vi "Write to Lights.vi"   [LabVIEW 2015]
uses:
  Common Code/Shooter State.ctl
  <vilib>/Rock Robotics/WPI/DriverStation/WPI_DriverStationRobotMode2.ctl
  <vilib>/Rock Robotics/WPI/DriverStation/WPI_DriverStationAllianceInfo.ctl
  Common Code/Utilities/TimeManager.vi
  Common Code/Change Detect.vi
  Common Code/Change Detect Boolean.vi
  Robot Global Data.vi
types:
  T1 = typedef "WPI_DriverStationAllianceInfo.ctl" = enum16{"Red", "Blue", "Invalid"}
  T2 = typedef "Shooter State.ctl" = enum16{"Idle", "Settle Ball", "Warmup", "Shooter Ready", "Shoot"}
  T3 = typedef "WPI_DriverStationRobotMode2.ctl" = enum16{"Autonomous Disabled", "Autonomous Enabled", "Teleop Disabled", "Teleop Enabled", "Disconnected", "Finish", "Test Disabled", "Test Enabled", "Emergency Stopped"}
  T4 = typedef "Shooter State Cluster.ctl" = cluster{"State":T2, "Left RPM":dbl, "Right RPM":dbl, "Shooter Ready?":bool, "Ball Loaded?":bool, "Current Angle":dbl, "Angle Motor Output":dbl, "Trigger Output":dbl, "Angle Ready?":bool, "RPM Ready?":bool, "Vision Ready?":bool, "Ball Loaded?":bool, "Mode":T5, "Shot Type":T6, "Pot Height":dbl, "Current Tripped Forward?":bool, "Current Tripped Backward?":bool, "Right Servo":i32, "Left Servo":i32, "IR Override":bool, "Intake Danger?":bool, "Intake Angle Ready?":bool}
  T5 = typedef "Shoot Modes Enum.ctl" = enum16{"Manual", "Auto"}
  T6 = typedef "Shot Type.ctl" = enum16{"Batter Shot", "Corner Shot", "Cleat Shot", "Vision Shot", "Deep Middle Shot"}
  T7 = typedef "WPI_AOChannelDevRef.ctl" = cluster{"DevStatus":errorcluster, "AO Channel":T8}
  T8 = typedef "WPI_AnalogOutputChannel.ctl" = enum8{"AO MXP 0", "AO MXP 1", "Invalid"}
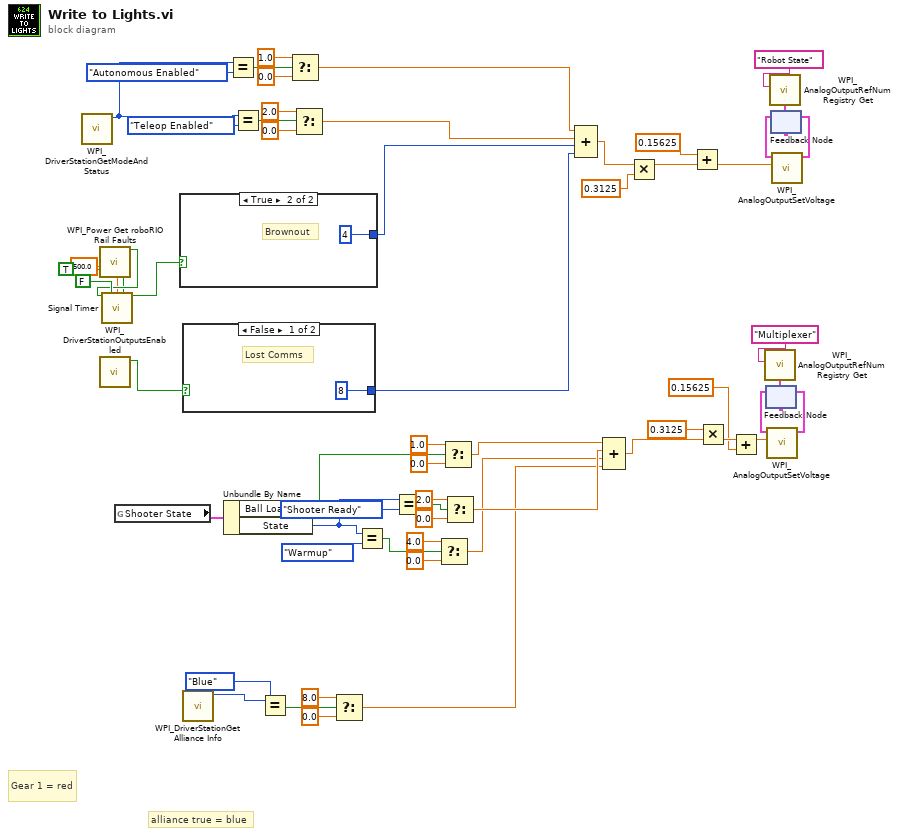
[diagram p0: block diagram]
diagram:
  # "alliance true = blue"
  # "Gear 1 = red"
  n1 = call <vilib>:"WPI_DriverStationGetModeAndStatus.vi"() -> ("Robot Mode"=w25:T3)  [unwired: 10 in, 1 out]
  n2 = call <vilib>:"WPI_Power Get roboRIO Rail Faults.vi"() -> ("Input Voltage Brown Out"=w50:bool)  [unwired: 10 in, 5 out]
  n3 = call <vilib>:"WPI_DriverStationOutputsEnabled.vi"() -> ("OutputsEnabled?"=w45:bool)  [unwired: 10 in, 1 out]
  n4 = call "Signal Timer.vi"("Input"=w50, "Edge"=FALSE, "Interval"=500.0, "Pull"=TRUE) -> ("Filtered Output"=w48:bool)  [unwired: 11 in]
  n5 = global read "Robot Global Data.vi" "Shooter State"() -> (w38:T4)
  n6 = case shown="True" w48 {
    tunnel: [_ 4] -> w44
    frame False {
    }
    frame True {
      # "Brownout"
    }
  }
  n7 = case shown="False" w45 {
    tunnel: [8 _] -> w43
    frame False {
      # "Lost Comms"
    }
    frame True {
    }
  }
  n8 = call <vilib>:"WPI_DriverStationGet Alliance Info.vi"() -> ("Alliance"=w7:T1)  [unwired: 10 in, 1 out]
  n9 = Unbundle By Name(w38) -> ("Ball Loaded?"=w35:bool, "State"=w36:T2)
  n10 = Equal?(x=w25, y=WPI_DriverStationRobotMode2."Autonomous Enabled") -> (x = y?=w23:bool)
  n11 = Equal?(x=w25, y=WPI_DriverStationRobotMode2."Teleop Enabled") -> (x = y?=w22:bool)
  n12 = Equal?(x=w7, y=WPI_DriverStationAllianceInfo."Blue") -> (x = y?=w5:bool)
  n13 = Select(t=1.0, s=w23, f=0.0) -> (s? t:f=w17:dbl)
  n14 = Select(t=2.0, s=w22, f=0.0) -> (s? t:f=w16:dbl)
  n15 = Select(t=8.0, s=w5, f=0.0) -> (s? t:f=w1:dbl)
  n16 = Equal?(x=w36, y=Shooter_State."Warmup") -> (x = y?=w29:bool)
  n17 = Equal?(x=w36, y=Shooter_State."Shooter Ready") -> (x = y?=w32:bool)
  n18 = Select(t=4.0, s=w29, f=0.0) -> (s? t:f=w13:dbl)
  n19 = Select(t=1.0, s=w35, f=0.0) -> (s? t:f=w15:dbl)
  n20 = Select(t=2.0, s=w32, f=0.0) -> (s? t:f=w14:dbl)
  n21 = Compound Arithmetic op=ADD(w17, w16, w44, w43) -> (w46:dbl)
  n22 = Compound Arithmetic op=ADD(w15, w14, w13, w1) -> (w12:dbl)
  n23 = Multiply(x=w46, y=0.3125) -> (x*y=w42:dbl)
  n24 = Add(x=0.15625, y=w42) -> (x+y=w40:dbl)
  n25 = Multiply(x=0.3125, y=w12) -> (x*y=w11:dbl)
  n26 = Add(x=w11, y=0.15625) -> (x+y=w9:dbl)
  n27 = call <vilib>:"WPI_AnalogOutputRefNum Registry Get.vi"("refnum name"="Multiplexer") -> ("AODeviceRef"=w54:T7)  [unwired: 9 in, 1 out]
  n28 = feedback #1(w54) -> (w53:T7)
  n29 = call <vilib>:"WPI_AnalogOutputSetVoltage.vi"("Voltage"=w9, "AODeviceRef"=w53) -> ("AODeviceRef"=w55:T7)  [unwired: 8 in, 1 out]
  n30 = feedback-in #1(w55) -> ()
  n31 = call <vilib>:"WPI_AnalogOutputRefNum Registry Get.vi"("refnum name"="Robot State") -> ("AODeviceRef"=w58:T7)  [unwired: 9 in, 1 out]
  n32 = feedback #2(w58) -> (w57:T7)
  n33 = call <vilib>:"WPI_AnalogOutputSetVoltage.vi"("Voltage"=w40, "AODeviceRef"=w57) -> ("AODeviceRef"=w59:T7)  [unwired: 8 in, 1 out]
  n34 = feedback-in #2(w59) -> ()
